vi "Andor_LoadAcqGraph.vi"(8 "ErrIn(No Err)":errorcluster caption="entrée d'erreur (pas d'erreur)") -> (0 "ErrOut":errorcluster caption="sortie d'erreur", 3 "ViRef":refnum<vi>)   [LabVIEW 2019]
panel:
  in  "AndorOpQ":refnum<queue>
  in  "AndorAcqQ":refnum<queue>
  out "Exécution:État":T1(ring)
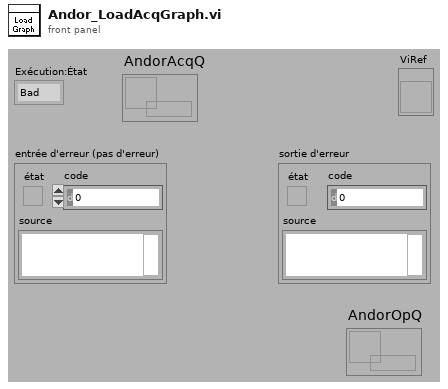
[diagram p1: front panel]
types:
  T1 = enum32{"Bad", "Idle", "Run top level", "Running"}
  T2 = enum16{"Répertoire du VI actuel", "Répertoire du parent 1", "Répertoire du parent 2", "Répertoire du parent 3"}
  T3 = enum32{"Invalid", "Standard", "Closed", "Hidden", "Minimized", "Maximized"}
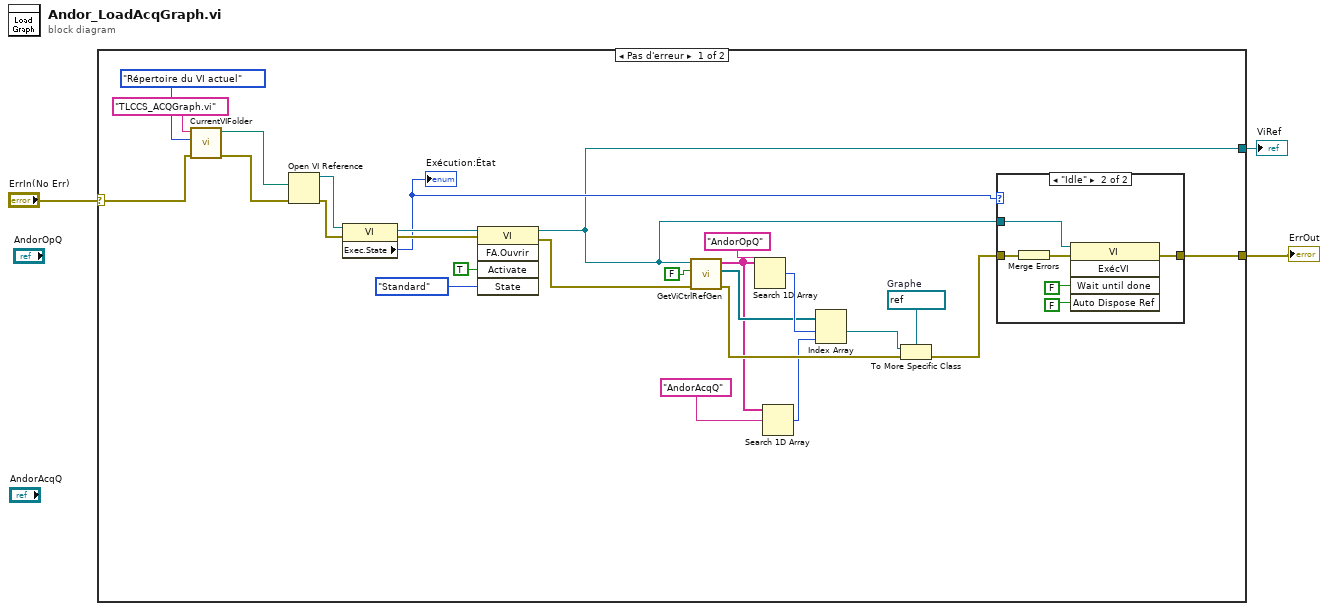
[diagram p0: block diagram]
diagram:
  n1 = case shown="Pas d'erreur" "ErrIn(No Err)" {
    selector: "ErrIn(No Err)" -> [w6 w37]
    tunnel: [w23 w37] -> w2
    tunnel: [w10 _] -> w1
    frame No Error {
      w25 = refnum<vi> refnum  # Graphe
      n2 = call <userlib>:"CurrentVIFolder.vi"("error in (no error)"=w6, "Source"=T2."Répertoire du VI actuel", "NomFichier"="TLCCS_ACQGraph.vi") -> ("error out"=w5:errorcluster, "Chemin"=w7:path)  [unwired: 6 in, 1 out]
      n3 = Open VI Reference(vi path=w7, error in (no error)=w5) -> (vi reference=w17:refnum<vi>, error out=w16:errorcluster)  [unwired: 4 in]
      n4 = property class="VI"(reference=w17, error in=w16) -> (reference out=w14:refnum<vi>, error out=w15:errorcluster, "Exec.State"=w13:T1)
      "Exécution:État" <- w13
      n5 = invoke class="VI" method="FA.Ouvrir"(reference=w14, error in=w15, "Activate"=TRUE ("Activer ?"), "State"=T3."Standard" ("État")) -> (reference out=w10:refnum<vi>, error out=w18:errorcluster)  [unwired: 1 in, 3 out]
      n6 = call <userlib>:"GetViCtrlRefGen.vi"("ErrorIn(No Error)"=w18, "InclTabCTrl"=FALSE, "VIRef"=w10) -> ("sortie d'erreur"=w21:errorcluster, "ControlsRefs"=w22:refnum<vi>[], "ControlsNames"=w9:string[])  [unwired: 6 in]
      n7 = Search 1D Array(1D array=w9, element="AndorOpQ" ("élément")) -> (index of element=w27:i32)  [unwired: 1 in]
      n8 = Search 1D Array(1D array=w9, element="AndorAcqQ" ("élément")) -> (index of element=w11:i32)  [unwired: 1 in]
      n9 = Index Array(array=w22, index #1=w27, index #2=w11) -> (element #1=w26:refnum<vi>)  [unwired: 1 out]
      n10 = To More Specific Class(target class=w25, reference=w26, error in=w21) -> (error out=w24:errorcluster)  [unwired: 1 out]
      n11 = case shown="\"Idle\"" w13 {
        tunnel: w24 -> [w30 w34]
        tunnel: [w30 w32] -> w23
        tunnel: w10 -> [_ w31]
        frame "Running", Default {
        }
        frame "Idle" {
          n12 = Merge Errors(w34) -> (w33:errorcluster)
          n13 = invoke class="VI" method="ExécVI"(reference=w31, error in=w33, "Wait until done"=FALSE ("Attendre la fin"), "Auto Dispose Ref"=FALSE ("Supprimer la référence automatiquement")) -> (error out=w32:errorcluster)  [unwired: 1 in, 4 out]
        }
      }
    }
    frame Error {
    }
  }
  "ErrOut" <- w2
  "ViRef" <- w1
